vi "GetVersion.vi"(8 "Error Input":errorcluster, 11 "LiteAgentSDK Input":refnum<k24>) -> (0 "Error Output":errorcluster, 2 "Version":string, 3 "LiteAgentSDK Output":refnum<k24>)   [LabVIEW 2017, in "LiteAgentSDK.lvlib"]
uses:
  LiteAgentSDK.lvlib
  C:/Users/Jan/Projects/LiteAgentSDK-LabVIEW/Source/Bin/LiteAgentSDK.LabVIEW.dll
  Bin/LiteAgentSDK.LabVIEW.dll
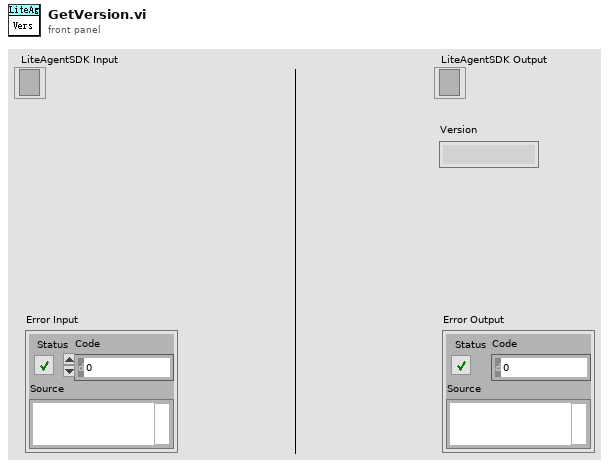
[diagram p1: front panel]
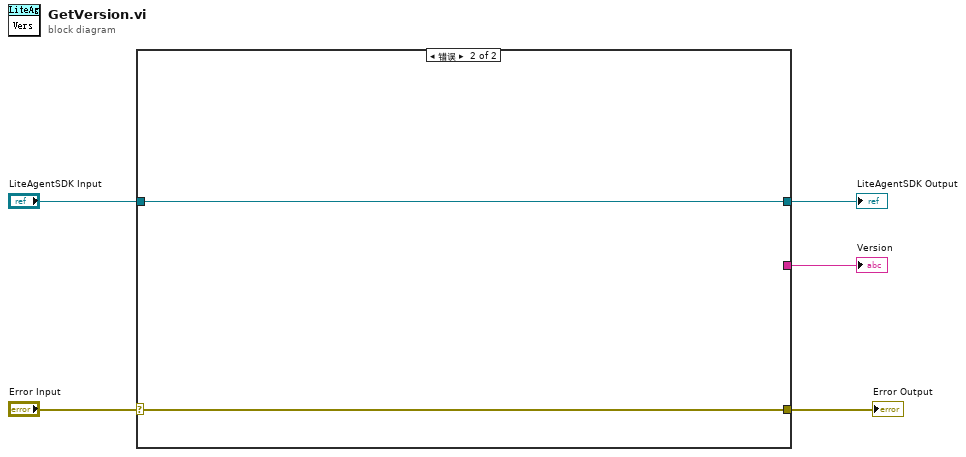
[diagram p0: block diagram]
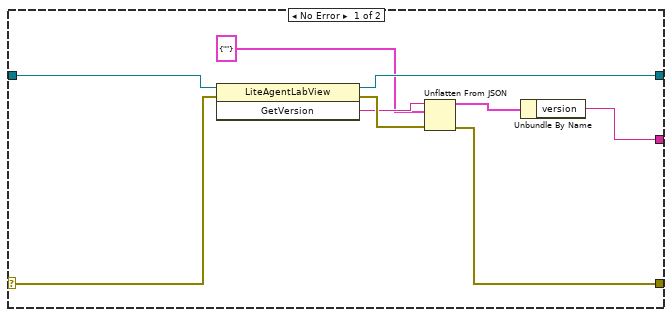
[diagram p2: hidden frame]
diagram:
  n1 = case shown="错误" "Error Input" {
    selector: "Error Input" -> [w13 w15]
    tunnel: "LiteAgentSDK Input" -> [w14 w16]
    tunnel: [w12 w16] -> w2
    tunnel: [w10 w15] -> w4
    tunnel: [w6 _] -> w1
    frame No Error {
      n2 = invoke on="调用节点" class="LiteAgentLabView" method="GetVersion"(reference=w14, error in=w13) -> (reference out=w12:refnum<k24>, error out=w11:errorcluster, "GetVersion"=w9:string)  [unwired: 1 in]
      n3 = Unflatten From JSON(JSON string=w9, type and defaults=cluster{"version":string} {"version"=""} ("VersionModel"), error in (no error)=w11) -> (value=w7:cluster{"version":string}, error out=w10:errorcluster)  [unwired: 4 in]
      n4 = Unbundle By Name(w7) -> ("version"=w6:string)
    }
    frame Error {
    }
  }
  "Error Output" <- w4
  "LiteAgentSDK Output" <- w2
  "Version" <- w1
